vi "Set Acquisition Rate.vi"() -> ()   [LabVIEW 2020]
uses:
  _libraries/Startup Processes/_typedefs/Subpanel Names.ctl
  toolbox/Standard Signalling/not_Generic Named Notifier/not_Generic Named Notifier.lvlib
  _ude/Set Acquisition Rate/Set Acquisition Rate.lvlib
  _libraries/Startup Processes/Startup Processes.lvlib
panel:
  out "Raw Response":variant
  out "Error Out":errorcluster
  in  "Acquisition Rate":i32
  in  "Plugin Names":T1
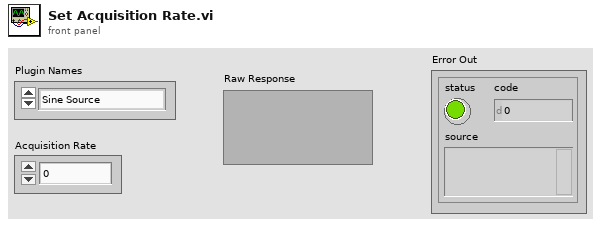
[diagram p1: front panel]
types:
  T1 = typedef "Startup Processes.lvlib/Subpanel Names.ctl" = enum16{"Sine Source", "Ramp Source", "Hen House TC", "Dog House TC", "Out House TC"}
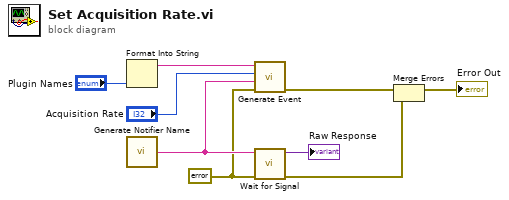
[diagram p0: block diagram]
diagram:
  w1 = errorcluster {"status"=FALSE, "code"=0, "source"=""} ("Error In")
  n1 = Format Into String("Plugin Names") -> (resulting string=w5:string)  [unwired: 3 in, 1 out]
  n2 = call "Generate Notifier Name.vi"() -> ("Notifier Name"=w3:string)
  n3 = call "Generate Event.vi"("Error In"=w1, "Response Notifier"=w3, "Sample Period"="Acquisition Rate", "Source Name"=w5) -> ("Error Out"=w2:errorcluster)  [unwired: 3 in]
  n4 = call "Wait for Signal.vi"("Error In"=w1, "Notifier Name"=w3) -> ("Error Out"=w6:errorcluster, "Signal Data"=→"Raw Response":variant)  [unwired: 4 in]
  n5 = Merge Errors(w2, w6) -> (→"Error Out":errorcluster)
